vi "Append Front Panel Image to Report (refnum).vi"(0 "report in":refnum<class "NI_report.lvclass">, 1 "alignment (default)":T2, 2 "image format (jpeg)":enum32{"PNG", "JPEG", "GIF"}(ring)=enum."JPEG", 5 "VI":refnum<vi>, 9 "description":string, 11 "error in (no error)":errorcluster, 12 "visible area only?":bool, 13 "MS Office parameters":T1) -> (4 "report out":refnum<class "NI_report.lvclass">, 6 "VI out":refnum<vi>, 8 "start out (Word)":i32, 10 "end out (Word)":i32, 15 "error out":errorcluster)   [LabVIEW 2017, in "NI_ReportGenerationCore.lvlib"]
doc: "Creates an image of the front panel of the VI you specify in <B>VI</B> and appends it to a report. Wire data to the <B>VI</B> input to determine the polymorphic instance to use or manually select the instance."
uses:
  <vilib>/Utility/NIReport.llb/NI_ReportGenerationCore.lvlib
  <vilib>/Utility/NIReport.llb/NI_report.lvclass
  <vilib>/Utility/NIReport.llb/HTML Report Image Alignment.ctl
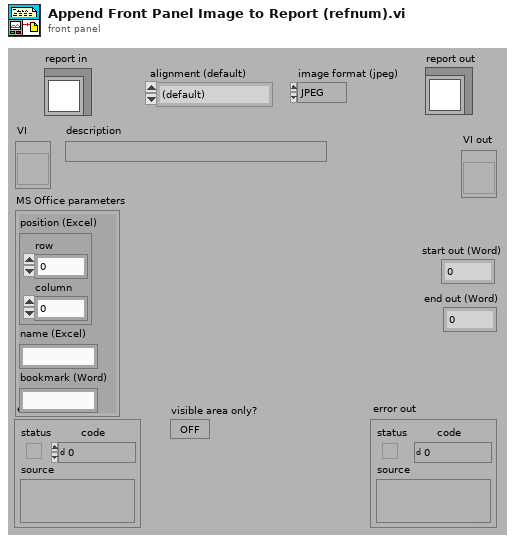
[diagram p1: front panel]
types:
  T1 = cluster{"position (Excel)":cluster{"row":i32, "column":i32}, "name (Excel)":string, "bookmark (Word)":string}
  T2 = typedef "NI_ReportGenerationCore.lvlib/HTML Report Image Alignment.ctl" = enum16{"(default)", "LEFT", "RIGHT", "TOP", "TEXTTOP", "MIDDLE", "ABSMIDDLE", "BASELINE", "BOTTOM", "ABSBOTTOM"}
  T3 = typedef "imagedata.ctl" = cluster{"image type":i32, "image depth":i32, "image":u8[], "mask":u8[], "colors":u32[], "Rectangle":cluster{"left":i16, "top":i16, "right":i16, "bottom":i16}}
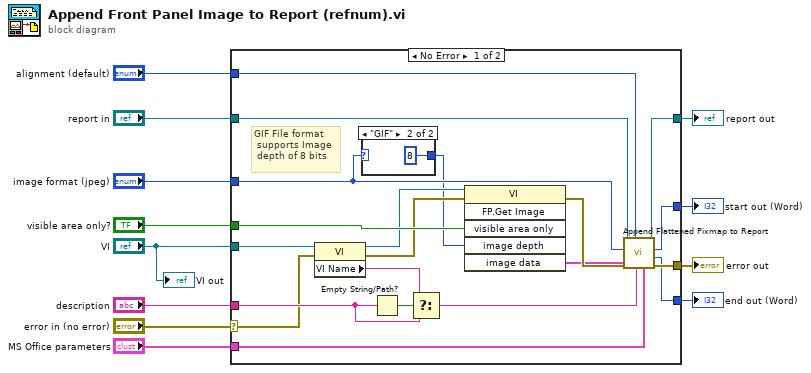
[diagram p0: block diagram]
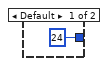
[diagram p2: hidden frame]
diagram:
  n1 = case shown="No Error" "error in (no error)" {
    selector: "error in (no error)" -> [w22 w36]
    tunnel: "description" -> [w32 _]
    tunnel: "visible area only?" -> [w31 _]
    tunnel: "VI" -> [w30 _]
    tunnel: "image format (jpeg)" -> [w18 _]
    tunnel: [w23 w36] -> w6
    tunnel: [w14 w35] -> w7
    tunnel: "alignment (default)" -> [w25 _]
    tunnel: "report in" -> [w13 w35]
    tunnel: "MS Office parameters" -> [w20 _]
    tunnel: [w16 _] -> w2
    tunnel: [w15 _] -> w1
    frame No Error {
      # "GIF File format\n supports Image\n depth of 8 bits"
      n2 = property class="VI"(reference=w30, error in=w22) -> (reference out=w27:refnum<vi>, error out=w26:errorcluster, "VI Name"=w28:string)
      n3 = case shown="\"GIF\"" w18 {
        tunnel: [24 ("image depth") 8 ("image depth")] -> w17
        frame Default {
        }
        frame "GIF" {
        }
      }
      n4 = Empty String/Path?(string/path=w32) -> (empty?=w29:bool)
      n5 = Select(t=w28, s=w29, f=w32) -> (s? t:f=w21:string)
      n6 = invoke class="VI" method="FP.Get Image"(reference=w27, error in=w26, "visible area only"=w31, "image depth"=w17) -> (error out=w24:errorcluster, "image data"=w19:T3)  [unwired: 2 in, 4 out]
      n7 = call <vilib>:"Append Flattened Pixmap to Report.vi"("MS Office parameters"=w20, "caption or alt string"=w21, "alignment (default)"=w25, "error in (no error)"=w24, "image data"=w19, "image format (jpeg)"=w18, "report in"=w13) -> ("error out"=w23:errorcluster, "end out (word)"=w15:i32, "start out (word)"=w16:i32, "report out"=w14:refnum<class "NI_report.lvclass">)  [unwired: 1 in]
    }
    frame Error {
    }
  }
  "error out" <- w6
  "report out" <- w7
  "start out (Word)" <- w2
  "end out (Word)" <- w1
  "VI out" <- "VI"
